vi "Read SubVIs.vi"(9 "PyConvBD in":refnum<class "PyConvBD.lvclass">) -> (3 "PyConvBD out":refnum<class "PyConvBD.lvclass">, 4 "SubVIs":variant)   [LabVIEW 2014, in "Raspberry Pi Compatible Compiler for LabVIEW.lvlib" / "PyConvBD.lvclass"]
uses:
  PyConvBD.lvclass
  PyConvBD.lvclass/PyConvBD.ctl
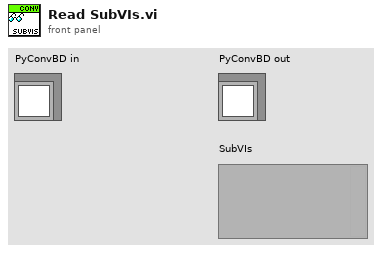
[diagram p1: front panel]
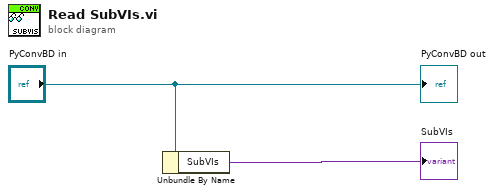
[diagram p0: block diagram]
diagram:
  n1 = Unbundle By Name("PyConvBD in") -> ("SubVIs"=→"SubVIs":variant)
  "PyConvBD out" <- "PyConvBD in"
